vi "applyDM_and_acqTIFF_mCMD.vi"(0 "EMCCD trigger port":tag="Dev1/port0/line0", 1 "WavefrontCorrector in":refnum<class "WavefrontCorrector.lvclass">, 3 "Absolute Positions":T1, 5 "exp and readout time (ms)":dbl, 7 "CMD Num":i32, 9 "Img Num":i32, 11 "error in (no error)":errorcluster, 12 "strPath":string="_groundtruth_", 13 "Clean Spooling":bool=TRUE, 14 "strPalette":string="C:\\Program Files\\Andor SOLIS\\GREY.PAL") -> (4 "WavefrontCorrector out":refnum<class "WavefrontCorrector.lvclass">, 15 "error out":errorcluster)   [LabVIEW 2018]
uses:
  <userlib>/WaveKit.lib/Classes/WavefrontCorrector/WavefrontCorrector.lvclass
  <vilib>/Analysis/Matrix/Datatypes/RealMatrix.ctl
  <vilib>/Analysis/Matrix/NI_Matrix.lvlib
panel:
  # "Default settings"
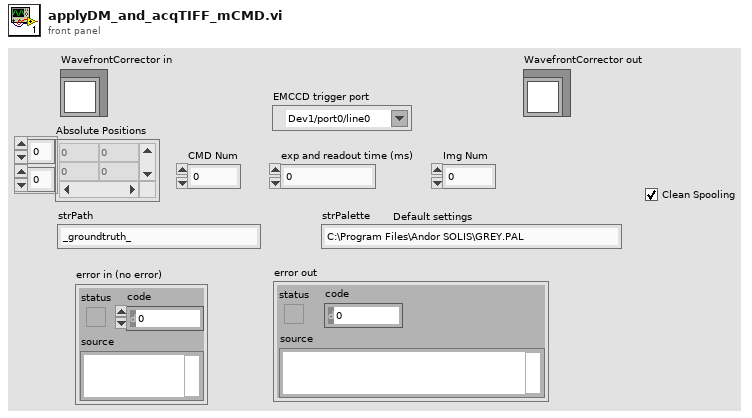
[diagram p1: front panel]
types:
  T1 = typedef "NI_Matrix.lvlib/RealMatrix.ctl" = dbl[][]
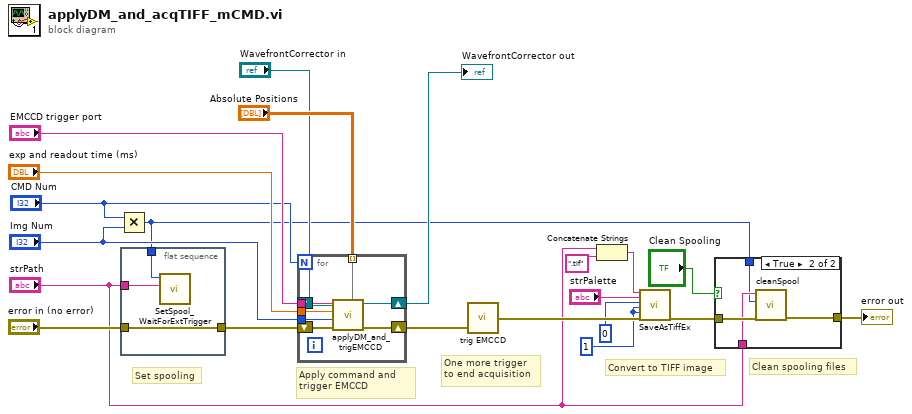
[diagram p0: block diagram]
diagram:
  w14 = 1
  # "Apply command and \ntrigger EMCCD"
  # "Set spooling"
  # "Clean spooling files"
  # "Convert to TIFF image"
  # "One more trigger\nto end acquisition"
  n1 = Multiply(x="CMD Num", y="Img Num") -> (x*y=w1:i32)
  n2 = flat-sequence {
    tunnel: "strPath" -> [w24]
    tunnel: w1 -> [w23]
    tunnel: "error in (no error)" -> [w22]
    tunnel: [w22] -> w11
    frame #0 {
      n3 = call "SetSpool_WaitForExtTrigger.vi"("path and name"=w24, "Kinetic Series"=w23) -> ()  [unwired: 10 in]
    }
  }
  n4 = for {
    N: "CMD Num" -> [_]
    tunnel: "EMCCD trigger port" -> [w32]
    tunnel: "Absolute Positions" -> [w31] mode=indexing
    tunnel: "exp and readout time (ms)" -> [w29]
    tunnel: "Img Num" -> [w25]
    shift-right: [w27] -> w10
    shift-left: "WavefrontCorrector in" -> [w30]
    shift-right: [w26] -> w9
    shift-left: w11 -> [w28]
    n5 = call "applyDM_and_trigEMCCD.vi"("Absolute Positions"=w31, "WavefrontCorrector in"=w30, "error in (no error)"=w28, "Trig Num"=w25, "exp and readout time (ms)"=w29, "EMCCD trigger port"=w32) -> ("error out"=w26:errorcluster, "WavefrontCorrector out"=w27:refnum<class "WavefrontCorrector.lvclass">)  [unwired: 4 in]
  }
  "WavefrontCorrector out" <- w10
  n6 = call "trig EMCCD.vi"("error in (no error)"=w9) -> ("error out"=w17:errorcluster)  [unwired: 2 in]
  n7 = Concatenate Strings("strPath", ".tif") -> (w16:string)
  n8 = call <userlib>:"SaveAsTiffEx.vi"("path"=w16, "palette"="strPalette", "position"=0, "type"=w14, "mode"=w14, "error in (no error)"=w17) -> ("error out"=w7:errorcluster)  [unwired: 12 in, 1 out]
  n9 = case shown="True" "Clean Spooling" {
    tunnel: w7 -> [w33 w37]
    tunnel: [w33 w36] -> w6
    tunnel: "strPath" -> [_ w35]
    tunnel: w1 -> [_ w34]
    frame False {
    }
    frame True {
      n10 = call "cleanSpool.vi"("error in (no error)"=w37, "Total Img Num"=w34, "strPath"=w35) -> ("error out"=w36:errorcluster)  [unwired: 8 in]
    }
  }
  "error out" <- w6
